vi "PC_sum_array.vi"(8 "error in (no error)":errorcluster, 11 "waveform in":waveform(dbl)) -> (0 "error out":errorcluster, 3 "Numeric":dbl)   [LabVIEW 2020]
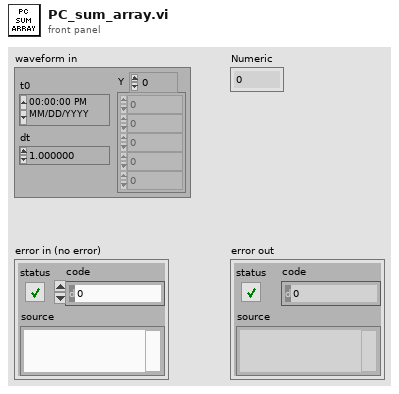
[diagram p1: front panel]
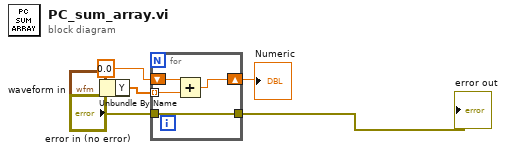
[diagram p0: block diagram]
diagram:
  n1 = Unbundle By Name("waveform in") -> ("Y"=w3:dbl[])
  n2 = for {
    shift-right: [w8] -> w4
    shift-left: 0.0 -> [w10]
    tunnel: w3 -> [w9] mode=indexing
    tunnel: "error in (no error)" -> [w7]
    tunnel: [w7] -> w6
    n3 = Add(x=w10, y=w9) -> (x+y=w8:dbl)
  }
  "error out" <- w6
  "Numeric" <- w4
